vi "PD250 - PWM.vi"(7 "Board Selector":T1, 9 "HMP4040_IN":refnum<visa-resource-name>, 11 "HMP4040 Channel Settings":T2={"CH1 Voltage"=24.0, "CH1 Current"=1.0, "CH1 Output"=TRUE, "CH2 Voltage"=24.0, "CH2 Current"=1.0, "CH2 Output"=TRUE, "CH3 Voltage"=24.0, "CH3 Current"=1.0, "CH3 Output"=TRUE, "CH4 Voltage"=24.0, "CH4 Current"=1.0, "CH4 Output"=TRUE, "Master Output"=TRUE} {"CH4 Current" format="%.3f"; "CH4 Voltage" format="%.3f"; "CH3 Current" format="%.3f"; "CH3 Voltage" format="%.3f"; "CH2 Current" format="%.3f"; "CH2 Voltage" format="%.3f"; "CH1 Current" format="%.3f"; "CH1 Voltage" format="%.3f"}) -> (0 "error out":errorcluster, 1 "Inactive Legs":dbl[](array[numeric])=[2.0], 2 "Active Legs":dbl[](array[numeric])=[2.0], 3 "ControlBoard OUT":refnum<visa-resource-name>)   [LabVIEW 2022 SP3]
uses:
  HMP4000 Communication/HMP4040_ChannelControl.ctl
  Serial Board Com/Board Select.ctl
  <vilib>/DAQmx/read.llb/DAQmx Read (Analog 1D Wfm NChan NSamp).vi
  <vilib>/DAQmx/miscellaneous.llb/DAQmx Fill In Error Info.vi
panel:
  in  "error in (no error) 2":errorcluster
  out "Duty Cycle VISA Write":string[](array[string])
  out "Analysis Leg":i32
  out "Waveforms":T3
  out "Active Leg":i32
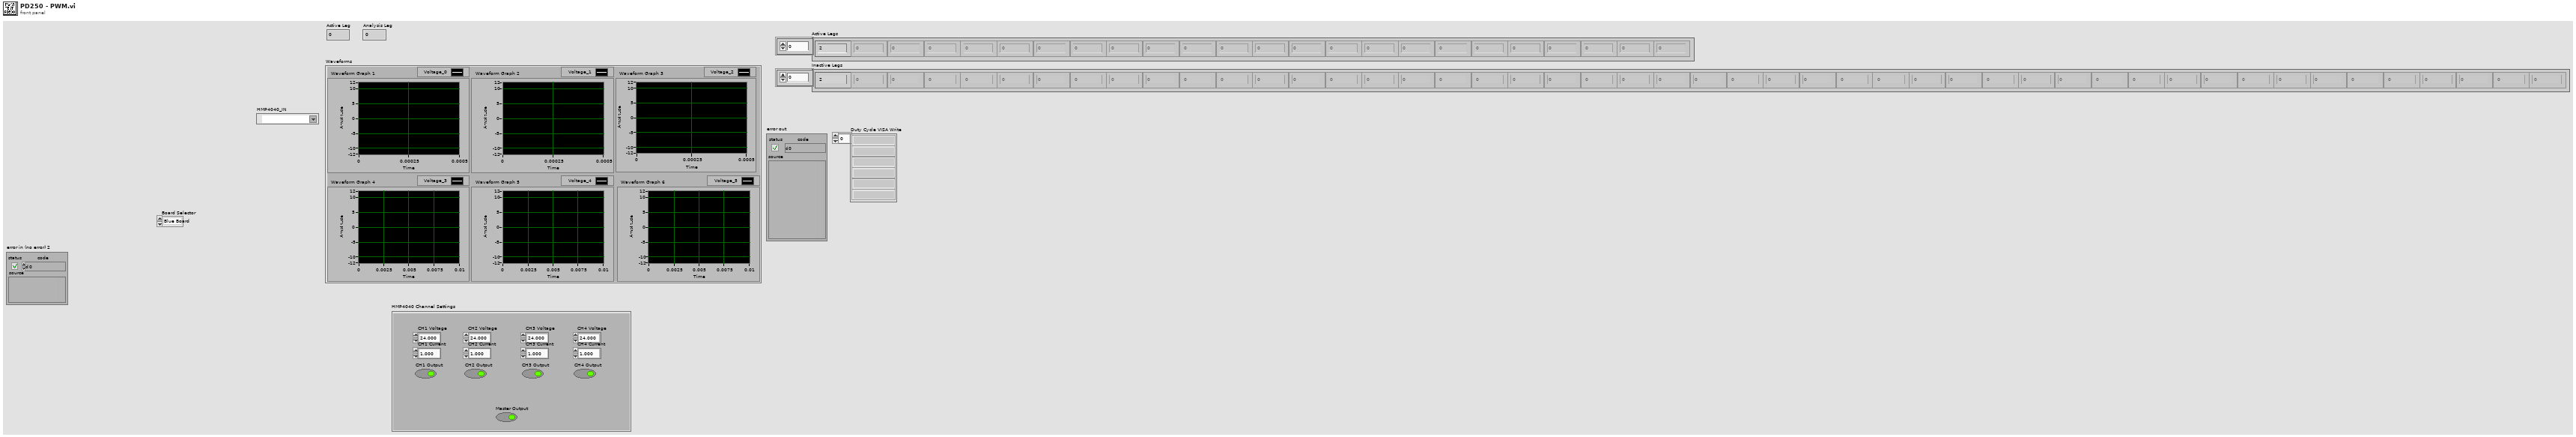
[diagram p1: front panel]
types:
  T1 = typedef "Board Select.ctl" = enum16{"Blue Board", "Green Board"}
  T2 = typedef "HMP4040_ChannelControl.ctl" = cluster{"CH1 Voltage":dbl, "CH1 Current":dbl, "CH1 Output":bool, "CH2 Voltage":dbl, "CH2 Current":dbl, "CH2 Output":bool, "CH3 Voltage":dbl, "CH3 Current":dbl, "CH3 Output":bool, "CH4 Voltage":dbl, "CH4 Current":dbl, "CH4 Output":bool, "Master Output":bool}
  T3 = cluster{"Waveform Graph 1":waveform(dbl), "Waveform Graph 2":waveform(dbl), "Waveform Graph 3":waveform(dbl), "Waveform Graph 4":waveform(dbl), "Waveform Graph 5":waveform(dbl), "Waveform Graph 6":waveform(dbl)}
  T4 = cluster{"data[0]":waveform(dbl), "data[1]":waveform(dbl), "data[2]":waveform(dbl), "data[3]":waveform(dbl), "data[4]":waveform(dbl), "data[5]":waveform(dbl)}
  T5 = typedef "NI_Matrix.lvlib/RealMatrix.ctl" = dbl[][]
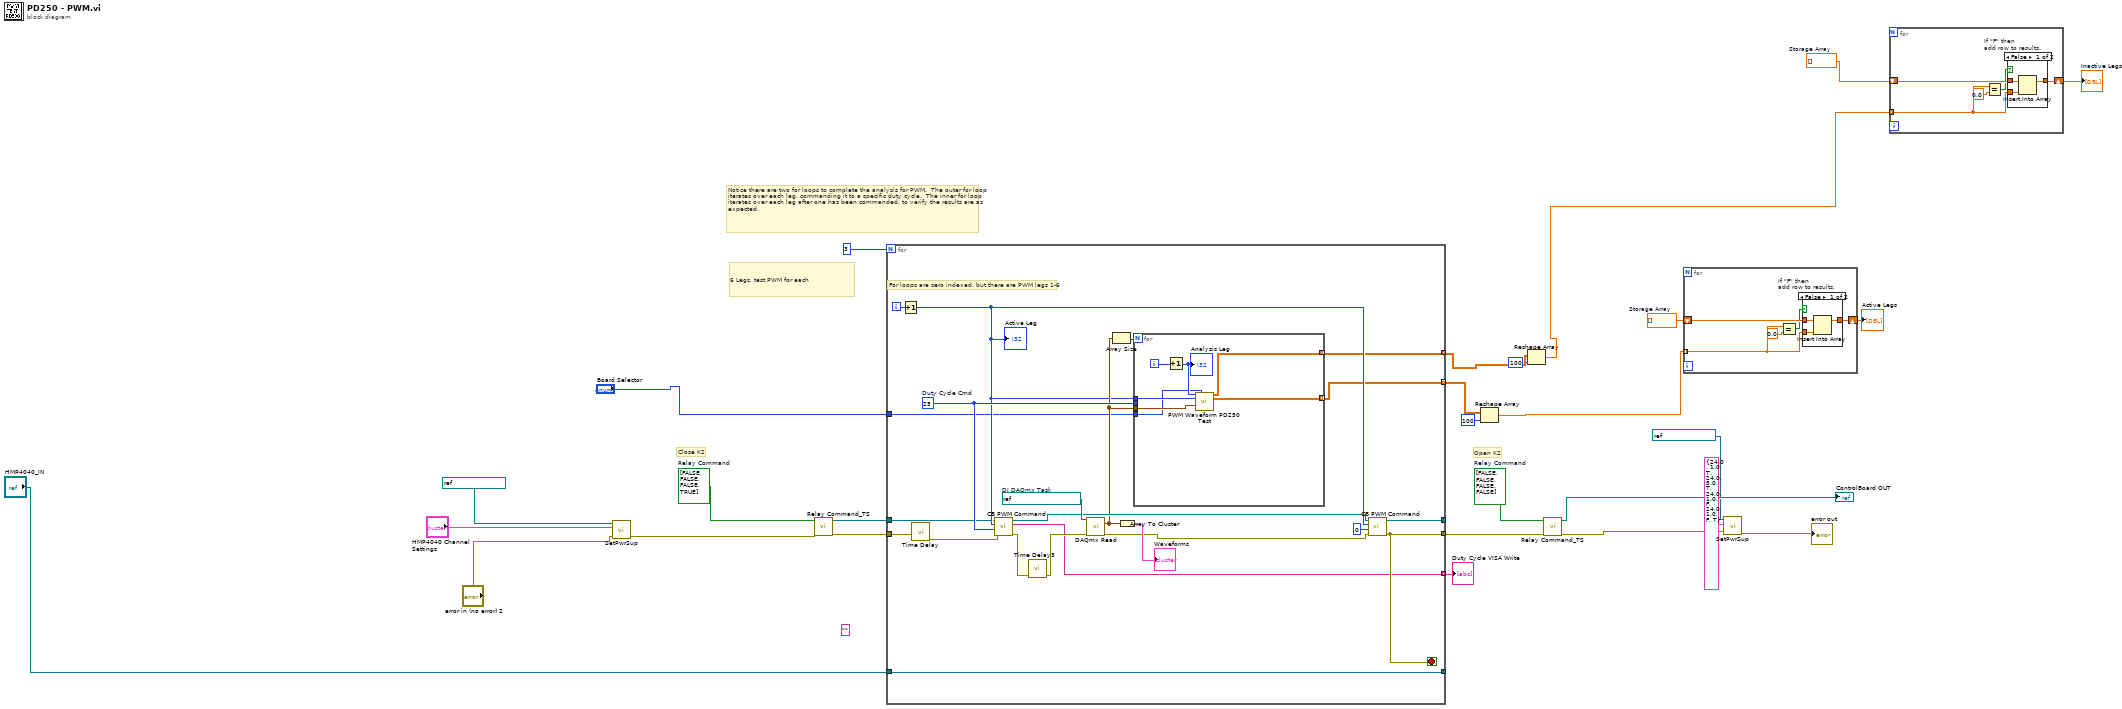
[diagram p0: block diagram]
diagram:
  w3 = dbl[] []  # Storage Array
  w6 = dbl[] []  # Storage Array
  w21 = bool[] [FALSE, FALSE, FALSE, TRUE]  # Relay Command
  w11 = bool[] [FALSE, FALSE, FALSE, FALSE]  # Relay Command
  (unwired) ""
  # "Close K2"
  # "Open K2"
  # "Notice there are two for loops to complete the analysis for PWM.  The outer for loop iterates over each leg, commanding it to a specific duty cycle.  The inner for loop iterates over each leg after one has been commanded, to verify the results are as expected."
  # "6 Legs, test PWM for each"
  n1 = call "SetPwrSup.vi"("error in (no error)"="error in (no error) 2", "HMP4040 Channel Settings"="HMP4040 Channel Settings", "HMP4040 IN"=refnum<visa-resource-name> "HMP4040_FTS2" ("VISA resource name")) -> ("error out"=w17:errorcluster)  [unwired: 7 in, 1 out]
  n2 = call "Relay Command_TS.vi"("error in (no error)"=w17, "Relay Command"=w21) -> ("error out"=w23:errorcluster, "VISA Refnum out"=w25:refnum<visa-resource-name>)  [unwired: 8 in]
  n3 = for {
    N: 3 -> [_]
    tunnel: [w45] -> _
    tunnel: "HMP4040_IN" -> [w45]
    tunnel: [w44] -> w27
    tunnel: [w40] -> _
    tunnel: w23 -> [w33]
    tunnel: w25 -> [w38]
    tunnel: [w35] -> w22 mode=indexing
    tunnel: "Board Selector" -> [w34]
    tunnel: [w31] -> w10 mode=indexing
    tunnel: [w30] -> w8 mode=indexing
    i -> [w46]
    stop <- w44 stop-if-true
    w47 = 25  # Duty Cycle Cmd
    w50 = refnum<k21> "FTS2_PWMInput_DG"  # DI DAQmx Task
    # "For loops are zero indexed, but there are PWM legs 1-6"
    n4 = Increment(x=w46) -> (x+1=w39:i32)
    "Active Leg" <- w39
    n5 = call "Time Delay"("error in (no error)"=w33) -> ("error out"=w32:errorcluster)  [unwired: 10 in]
    n6 = call "CB PWM Command.vi"("error in (no error)"=w32, "Duty Cycle"=w47, "Leg"=w39, "VISA Refnum in"=w38) -> ("error out"=w37:errorcluster, "read buffer"=w35:string, "VISA Refnum out"=w48:refnum<visa-resource-name>)  [unwired: 5 in]
    n7 = call "Time Delay3"("error in (no error)"=w37) -> ("error out"=w36:errorcluster)  [unwired: 10 in]
    n8 = call-poly <vilib>:"DAQmx Read.vi"("task/channels in"=w50, "error in"=w36) -> ("data"=w41:waveform(dbl)[], "error out"=w29:errorcluster)  [unwired: 11 in, 1 out]
    n9 = Array Size(array=w41) -> (size(s)=w42:i32)
    n10 = Array To Cluster(array=w41) -> (cluster=→"Waveforms":T4)
    n11 = for {
      N: w42 -> [_]
      tunnel: w47 -> [_]
      tunnel: w41 -> [w57]
      tunnel: w39 -> [w56]
      tunnel: w34 -> [w53]
      tunnel: [w52] -> w31 mode=indexing
      tunnel: [w51] -> w30 mode=indexing
      i -> [w55]
      n12 = Increment(x=w55) -> (x+1=w54:i32)
      "Analysis Leg" <- w54
      n13 = call "PWM Waveform PD250 Test.vi"("Analysis Leg"=w54, "Board Selector"=w53, "Active Leg"=w56, "Waveform"=w57) -> ("Inactive Values"=w52:T5, "Active Values"=w51:T5)  [unwired: 9 in, 1 out]
    }
    n14 = call "CB PWM Command.vi"("error in (no error)"=w29, "Duty Cycle"=0, "Leg"=w39, "VISA Refnum in"=w48) -> ("error out"=w44:errorcluster, "VISA Refnum out"=w40:refnum<visa-resource-name>)  [unwired: 5 in, 1 out]
  }
  "Duty Cycle VISA Write" <- w22
  n15 = Reshape Array(w8, 100 ("dimension size")) -> (w1:dbl[])
  n16 = Reshape Array(w10, 100 ("dimension size")) -> (w4:dbl[])
  n17 = call "Relay Command_TS.vi"("error in (no error)"=w27, "Relay Command"=w11) -> ("error out"=w14:errorcluster, "VISA Refnum out"=→"ControlBoard OUT":refnum<visa-resource-name>)  [unwired: 8 in]
  n18 = for {
    tunnel: w1 -> [w60] mode=indexing
    shift-right: [w61] -> w2
    shift-left: w3 -> [w62]
    n19 = Equal?(x=w60, y=0.0) -> (x = y?=w58:bool)
    n20 = case "If \"F\" then \nadd row to results." shown="False" w58 {
      tunnel: w62 -> [w65 w66]
      tunnel: w60 -> [w64 _]
      tunnel: [w63 w66] -> w61
      frame False {
        n21 = Insert Into Array(array=w65, new element=w64) -> (w63:dbl[])  [unwired: 1 in]
      }
      frame True {
      }
    }
  }
  "Active Legs" <- w2
  n22 = call "SetPwrSup.vi"("error in (no error)"=w14, "HMP4040 Channel Settings"=T2 {"CH1 Voltage"=24.0, "CH1 Current"=1.0, "CH1 Output"=TRUE, "CH2 Voltage"=24.0, "CH2 Current"=5.0, "CH2 Output"=TRUE, "CH3 Voltage"=24.0, "CH3 Current"=1.0, "CH3 Output"=FALSE, "CH4 Voltage"=24.0, "CH4 Current"=1.0, "CH4 Output"=FALSE, "Master Output"=TRUE}, "HMP4040 IN"=refnum<visa-resource-name> "HMP4040_FTS2" ("VISA resource name")) -> ("error out"=→"error out":errorcluster)  [unwired: 7 in, 1 out]
  n23 = for {
    tunnel: w4 -> [w69] mode=indexing
    shift-right: [w70] -> w5
    shift-left: w6 -> [w71]
    n24 = Equal?(x=w69, y=0.0) -> (x = y?=w67:bool)
    n25 = case "If \"F\" then \nadd row to results." shown="False" w67 {
      tunnel: w71 -> [w74 w75]
      tunnel: w69 -> [w73 _]
      tunnel: [w72 w75] -> w70
      frame False {
        n26 = Insert Into Array(array=w74, new element=w73) -> (w72:dbl[])  [unwired: 1 in]
      }
      frame True {
      }
    }
  }
  "Inactive Legs" <- w5
